vi "Initialize Sessions - 1Sess.vi"(6 "initialize and close session behavior":T2, 7 "simulate (F)":bool, 8 "error in":errorcluster, 9 "reset device (T)":bool=TRUE, 10 "topology name":T1="Configured Topology", 11 "session reservation in":refnum<class "Session Reservation.lvclass">) -> (0 "error out":errorcluster, 1 "channel list":string, 2 "session":refnum<class "Session Factory.lvclass">, 3 "session reservation out":refnum<class "Session Reservation.lvclass">)   [LabVIEW 2021, in "Session Management niSwitch.lvlib"]
doc: "Create the NI-Switch driver session from the <b>session reservation in</b>. Returns an error if more than one NI-Switch session has been reserved. Use \"Initialize Sesssions - NSess.vi\" for multiple sessions."
uses:
  Session Management niSwitch.lvlib
  <vilib>/Plug-In SDKs/Clients/Session Management V1/Session Reservation/Session Reservation.lvclass
  <vilib>/Plug-In SDKs/Clients/Session Management V1/Session Reservation/Initialize and Close Session Behavior.ctl
  Session Factory/Session Factory.lvclass
  C:/Program Files/National Instruments/LabVIEW 2021/vi.lib/Plug-In SDKs/Sessions/Instrument/ISession Factory/ISession Factory.lvclass
  <instrlib>/niSwitch/niSwitch.llb/niSwitch Topologies.ctl
  c5bc7267-7907-4e4e-a44f-7145a9a1ed21.vi
  <vilib>/Plug-In SDKs/Clients/Session Management V1/Session Reservation/Initialize Sessions with Retry.vi
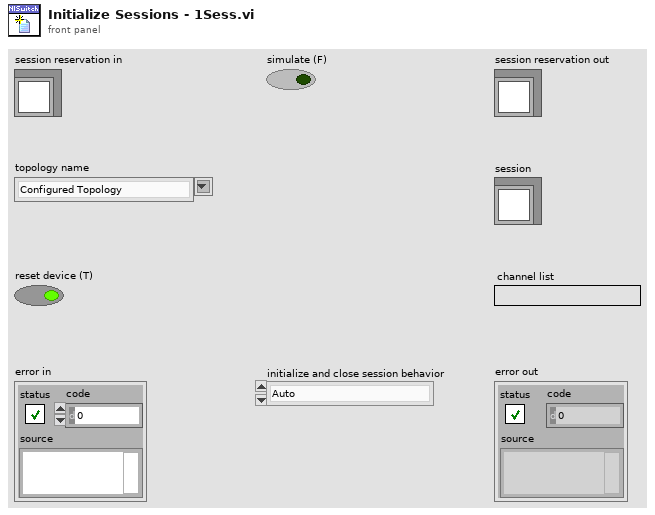
[diagram p1: front panel]
types:
  T1 = typedef "niSwitch Topologies.ctl" = string
  T2 = typedef "NI Session Management V1 Client.lvlib/Session Reservation.lvclass/Initialize and Close Session Behavior.ctl" = enum16{"Auto", "Initialize and Close", "Attach and Detach", "Initialize and Detach", "Attach and Close"}
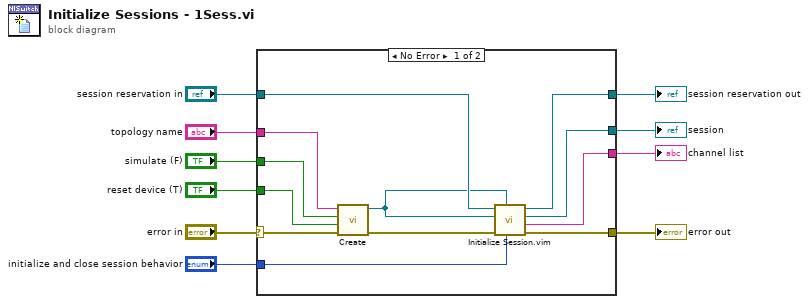
[diagram p0: block diagram]
diagram:
  n1 = case shown="No Error" "error in" {
    selector: "error in" -> [w16 w23]
    tunnel: [w20 w24] -> w10
    tunnel: "session reservation in" -> [w21 w24]
    tunnel: [w18 _] -> w9
    tunnel: [w17 _] -> w8
    tunnel: "initialize and close session behavior" -> [w15 _]
    tunnel: "topology name" -> [w14 _]
    tunnel: "simulate (F)" -> [w13 _]
    tunnel: "reset device (T)" -> [w12 _]
    tunnel: [w11 w23] -> w1
    frame No Error {
      n2 = call "Create.vi"("error in"=w16, "reset device"=w12, "simulate"=w13, "topology name"=w14) -> ("error out"=w22:errorcluster, "session factory out"=w19:refnum<class "Session Factory.lvclass">)  [unwired: 6 in]
      n3 = call "Initialize Session.vim"("initialize and close session behavior"=w15, "session type"=w19, "error in"=w22, "session factory"=w19, "session reservation in"=w21) -> ("error out"=w11:errorcluster, "channel list"=w17:string, "session"=w18:refnum<class "Session Factory.lvclass">, "session reservation out"=w20:refnum<class "Session Reservation.lvclass">)  [unwired: 3 in]
    }
    frame Error {
    }
  }
  "session reservation out" <- w10
  "error out" <- w1
  "session" <- w9
  "channel list" <- w8
